vi "Scale.vi"(8 "error in (no error)":errorcluster, 10 "Scale Factor":dbl, 11 "IScalable in":refnum<class "IScalable.lvclass">) -> (0 "error out":errorcluster, 3 "IScalable out":refnum<class "IScalable.lvclass">)   [LabVIEW 2021, in "Picture2D.lvlib" / "IScalable.lvclass"]
uses:
  IScalable.lvclass
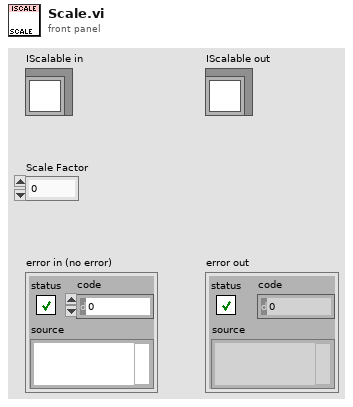
[diagram p1: front panel]
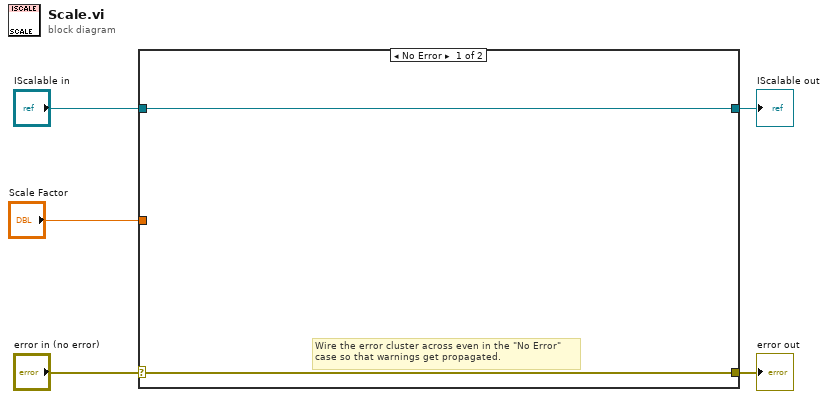
[diagram p0: block diagram]
diagram:
  n1 = case shown="No Error" "error in (no error)" {
    selector: "error in (no error)" -> [w6 w9]
    tunnel: [w6 w9] -> w4
    tunnel: [w7 w8] -> w2
    tunnel: "IScalable in" -> [w7 w8]
    tunnel: "Scale Factor" -> [_ _]
    frame No Error {
      # "Wire the error cluster across even in the \"No Error\"\ncase so that warnings get propagated."
    }
    frame Error {
    }
  }
  "error out" <- w4
  "IScalable out" <- w2
